vi "Constrain Image Size.vi"(6 "Local Data in":T1, 8 "error in (no error)":errorcluster) -> (0 "error out":errorcluster)   [LabVIEW 2024]
uses:
  Controls/RVHR - Local Data.ctl
  Controls/Test Cluster.ctl
  Controls/Excluded Information.ctl
  Controls/Language.ctl
  Controls/Device_Type.ctl
  <vilib>/Utility/miscctls.llb/LVRectTypeDef.ctl
  <vilib>/Utility/miscctls.llb/LVBoundsTypeDef.ctl
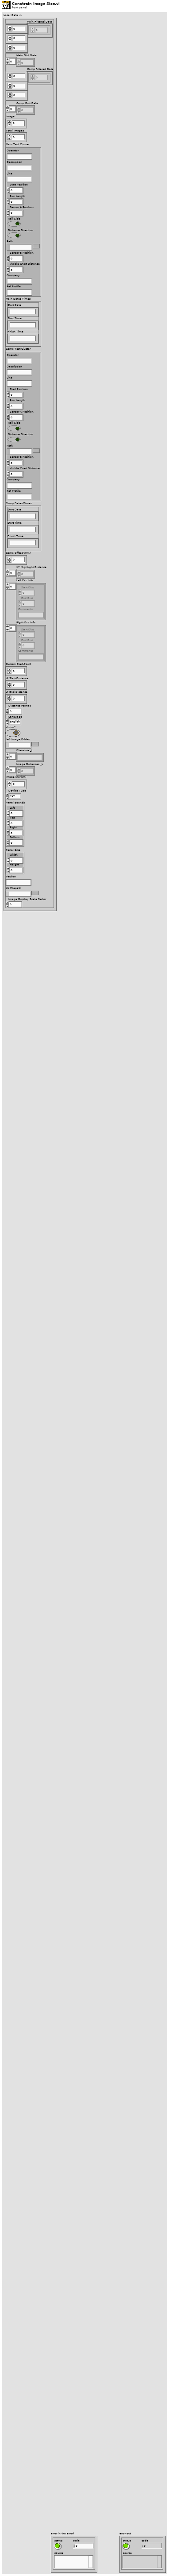
[diagram p1: front panel]
types:
  T1 = typedef "RVHR - Local Data.ctl" = cluster{"Main Filtered Data":dbl[][][], "Main Dist Data":dbl[], "Comp Filtered Data":dbl[][][], "Comp Dist Data":dbl[], "Image":u16, "Total Images":u16, "Main Test Cluster":T2, "Main Dates-Times":cluster{"Start Date":string, "Start Time":string, "Finish Time":string}, "Comp Test Cluster":T2, "Comp Dates-Times":cluster{"Start Date":string, "Start Time":string, "Finish Time":string}, "Comp Offset (mm)":i64, "XY Highlight Distance":dbl[], "Left Exc Info":T3[], "Right Exc Info":T3[], "Custom Start-Point":dbl, "UI Start-Distance":dbl, "UI End-Distance":dbl, "Distance Format":u8, "Language":T4, "Vision?":bool, "Left Image Folder":path, "Filename _L":string[], "Image Distances _L":dbl[], "Image Inc (km)":dbl, "Device Type":T5, "Panel Bounds":T6, "Panel Size":T7, "Version":string, "db Filepath":path, "Image Display Scale Factor":dbl}
  T2 = typedef "Test Cluster.ctl" = cluster{"Operator":string, "Description":string, "Line":string, "Start Position":dbl, "Run Length":dbl, "Sensor A Position":dbl, "Rail Side":bool, "Distance Direction":bool, "Path":path, "Sensor B Position":dbl, "Visible Chart Distance":dbl, "Company":string, "Ref Profile":string}
  T3 = typedef "Excluded Information.ctl" = cluster{"Start Dist":dbl, "End Dist":dbl, "Comments":string}
  T4 = typedef "Language.ctl" = enum16{"English", "Chinese", "German"}
  T5 = typedef "Device_Type.ctl" = enum16{"CAT", "Bi-CAT", "YRCA", "RCA", "RV-HR", "TV-HR"}
  T6 = typedef "LVRectTypeDef.ctl" = cluster{"Left":i16, "Top":i16, "Right":i16, "Bottom":i16}
  T7 = typedef "LVBoundsTypeDef.ctl" = cluster{"Width":u32, "Height":u32}
  T8 = typedef "IMAQ Image.ctl" = refnum<image>
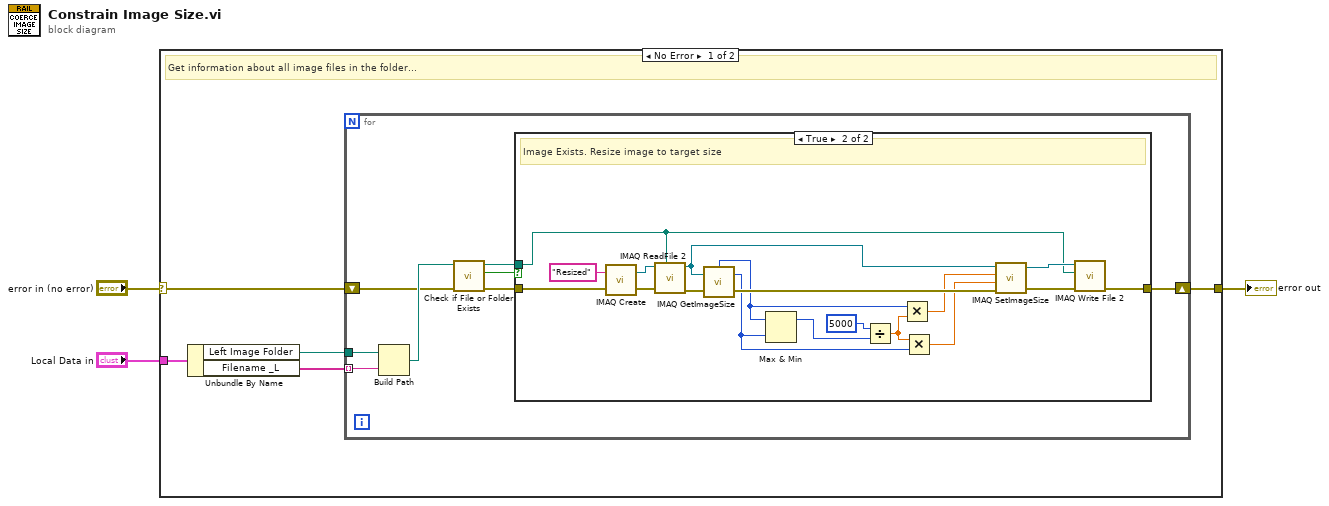
[diagram p0: block diagram]
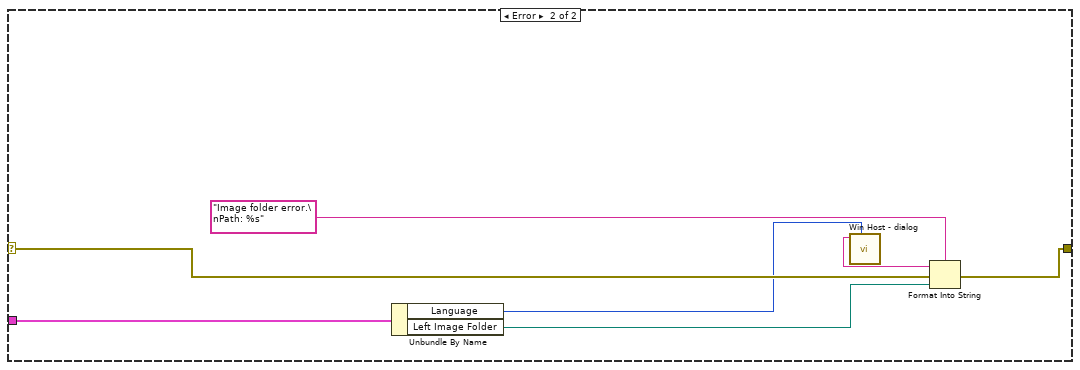
[diagram p3: hidden frame]
diagram:
  n1 = case shown="No Error" "error in (no error)" {
    selector: "error in (no error)" -> [w5 w40]
    tunnel: "Local Data in" -> [w8 w38]
    tunnel: [w4 w39] -> w1
    frame No Error {
      # "Get information about all image files in the folder..."
      n2 = Unbundle By Name(w8) -> ("Left Image Folder"=w6:path, "Filename _L"=w7:string[])
      n3 = for {
        tunnel: w7 -> [w16] mode=indexing
        tunnel: w6 -> [w15]
        shift-right: [w9] -> w4
        shift-left: w5 -> [w13]
        n4 = Build Path(base path=w15, name or relative path=w16) -> (appended path=w14:path)
        n5 = call <vilib>:"Check if File or Folder Exists.vi"("error in (no error)"=w13, "path"=w14) -> ("error out"=w12:errorcluster, "file or folder exists?"=w10:bool, "dup path"=w11:path)  [unwired: 7 in]
        n6 = case shown="True" w10 {
          tunnel: w11 -> [_ w18]
          tunnel: w12 -> [w17 w34]
          tunnel: [w17 w19] -> w9
          frame False {
          }
          frame True {
            # "Image Exists. Resize image to target size"
            n7 = call "IMAQ Create"("Image Name"="Resized", "error in (no error)"=w34) -> ("New Image"=w35:T8, "error out"=w33:errorcluster)  [unwired: 3 in]
            n8 = call "IMAQ ReadFile 2"("File Path"=w18, "error in (no error)"=w33, "Image"=w35) -> ("error out"=w31:errorcluster, "Image Out"=w30:T8)  [unwired: 4 in, 3 out]
            n9 = call "IMAQ GetImageSize"("Image"=w30, "error in (no error)"=w31) -> ("Y Resolution"=w26:i32, "X Resolution"=w28:i32, "error out"=w29:errorcluster)  [unwired: 2 in]
            n10 = Max & Min(x=w28, y=w26) -> (max(x,y)=w23:i32)  [unwired: 1 out]
            n11 = Divide(x=5000 ("Target Size"), y=w23) -> (x/y=w27:dbl)
            n12 = Multiply(x=w28, y=w27) -> (x*y=w25:dbl)
            n13 = Multiply(x=w27, y=w26) -> (x*y=w24:dbl)
            n14 = call "IMAQ SetImageSize"("error in (no error)"=w29, "Y Resolution"=w24, "X Resolution"=w25, "Image"=w30) -> ("error out"=w20:errorcluster, "Image Out"=w21:T8)  [unwired: 1 in]
            n15 = call-poly "IMAQ Write File 2"("error in (no error)"=w20, "File Path"=w18, "Image"=w21) -> ("error out"=w19:errorcluster)  [unwired: 7 in, 1 out]
          }
        }
      }
    }
    frame Error {
      n16 = Unbundle By Name(w38) -> ("Language"=w37:T4, "Left Image Folder"=w36:path)
      n17 = Format Into String(format string="Image folder error.\nPath: %s" ("Message"), error in=w40, w36) -> (resulting string=w41:string, error out=w39:errorcluster)  [unwired: 1 in]
      n18 = call "Win Host - dialog.vi"("Language"=w37, "Message"=w41) -> ()  [unwired: 8 in, 2 out]
    }
  }
  "error out" <- w1
